vi "GetWorldPosition.vi"(8 "group":i32, 10 "Snpx":refnum<k24>, 11 "error in":errorcluster) -> (0 "UserTool":i16, 1 "Cartesian position":T1, 2 "JointsPosition":dbl[](array[numeric]), 3 "error out":errorcluster)   [LabVIEW 2015, in "UnderAutomation.Fanuc.lvlib"]
uses:
  UnderAutomation.Fanuc.lvlib
  C:/Users/fg/Documents/Fanuc.vi/LabVIEW_2024/UnderAutomation.Fanuc/lib/UnderAutomation.Fanuc.dll
  LabVIEW_2024/UnderAutomation.Fanuc/lib/UnderAutomation.Fanuc.dll
panel:
  out "UserFrame":i16
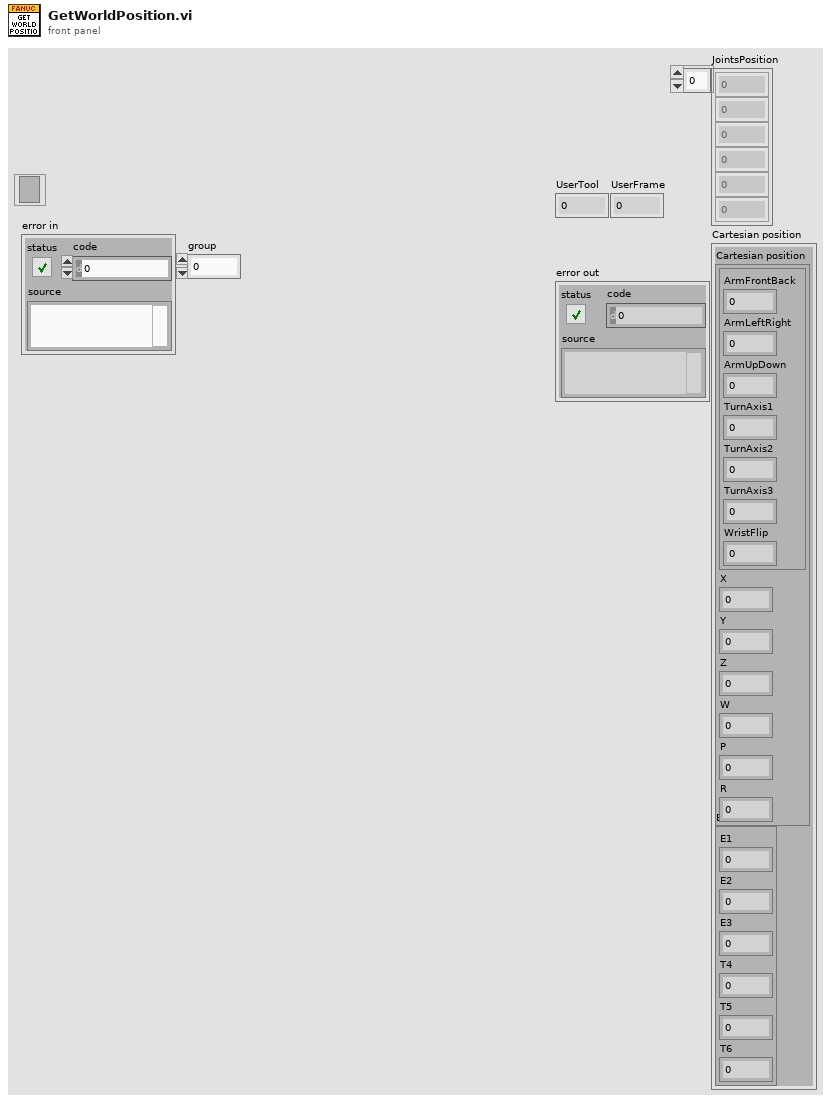
[diagram p1: front panel]
types:
  T1 = cluster{"Cartesian position":cluster{cluster{"ArmFrontBack":i32, "ArmLeftRight":i32, "ArmUpDown":i32, "TurnAxis1":i32, "TurnAxis2":i32, "TurnAxis3":i32, "WristFlip":i32}, "X":dbl, "Y":dbl, "Z":dbl, "W":dbl, "P":dbl, "R":dbl}, "Extension":cluster{"E1":dbl, "E2":dbl, "E3":dbl, "T4":i16, "T5":i16, "T6":i16}}
  T2 = cluster{"Configuration":cluster{"ArmFrontBack":i32, "ArmLeftRight":i32, "ArmUpDown":i32, "TurnAxis1":i32, "TurnAxis2":i32, "TurnAxis3":i32, "WristFlip":i32}, "X":dbl, "Y":dbl, "Z":dbl, "W":dbl, "P":dbl, "R":dbl}
  T3 = cluster{"E1":dbl, "E2":dbl, "E3":dbl, "E3":dbl, "E3":dbl, "E3":dbl}
  T4 = cluster{"Cartesian position":cluster{"Configuration":cluster{"ArmFrontBack":i32, "ArmLeftRight":i32, "ArmUpDown":i32, "TurnAxis1":i32, "TurnAxis2":i32, "TurnAxis3":i32, "WristFlip":i32}, "X":dbl, "Y":dbl, "Z":dbl, "W":dbl, "P":dbl, "R":dbl}, cluster{"E1":dbl, "E2":dbl, "E3":dbl, "E3":dbl, "E3":dbl, "E3":dbl}}
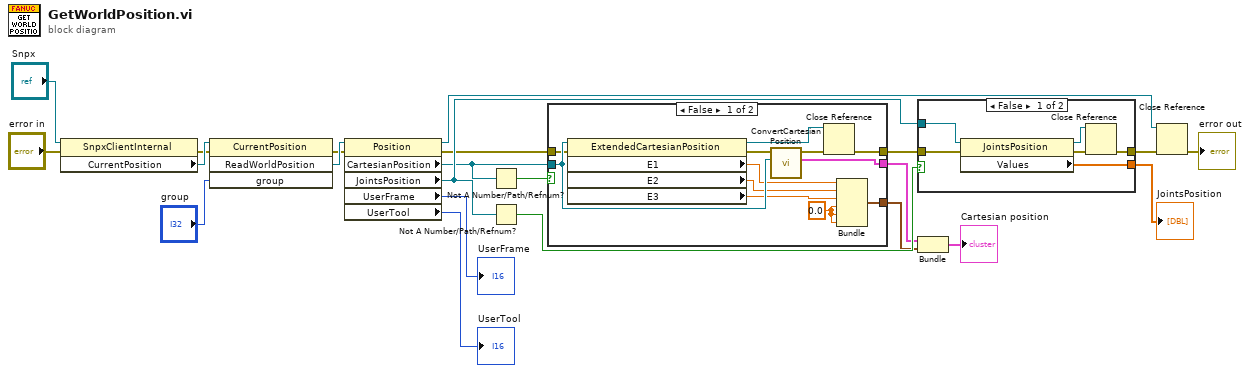
[diagram p0: block diagram]
diagram:
  n1 = property class="SnpxClientInternal"(reference="Snpx", error in="error in") -> (error out=w19:errorcluster, "CurrentPosition"=w20:refnum<k24>)  [unwired: 1 out]
  n2 = invoke class="CurrentPosition" method="ReadWorldPosition"(reference=w20, error in=w19, "group"="group") -> (error out=w3:errorcluster, "ReadWorldPosition"=w18:refnum<k24>)  [unwired: 1 in, 2 out]
  n3 = property class="Position"(reference=w18, error in=w3) -> (reference out=w17:refnum<k24>, error out=w6:errorcluster, "CartesianPosition"=w11:refnum<k24>, "JointsPosition"=w13:refnum<k24>, "UserFrame"=→"UserFrame":i16, "UserTool"=→"UserTool":i16)
  n4 = Not A Number/Path/Refnum?(number/path/refnum=w11) -> (NaN/Path/Refnum?=w10:bool)
  n5 = Not A Number/Path/Refnum?(number/path/refnum=w13) -> (NaN/Path/Refnum?=w14:bool)
  n6 = case shown="False" w10 {
    tunnel: w11 -> [w33 _]
    tunnel: [w34 _] -> w9
    tunnel: [w29 _] -> w8
    tunnel: w6 -> [w28 w35]
    tunnel: [w26 w35] -> w5
    frame False {
      w23 = 0.0 ("E3")
      n7 = property class="ExtendedCartesianPosition"(reference=w33, error in=w28) -> (reference out=w27:refnum<k24>, error out=w25:errorcluster, "E1"=w32:dbl, "E2"=w31:dbl, "E3"=w30:dbl)
      n8 = call "ConvertCartesianPosition.vi"("Cartesian position"=w33, "error in (no error)"=w25) -> ("Cartesian position"=w34:T2, "error out"=w24:errorcluster)  [unwired: 8 in]
      n9 = Close Reference(reference=w27, error in (no error)=w24) -> (error out=w26:errorcluster)
      n10 = Bundle("E1"=w32, "E2"=w31, "E3"=w30, "E3"=w23, "E3"=w23, "E3"=w23) -> (w29:T3)  [unwired: 1 in]
    }
    frame True {
    }
  }
  n11 = case shown="False" w14 {
    tunnel: w13 -> [w41 _]
    tunnel: [w40 _] -> w12
    tunnel: w5 -> [w37 w42]
    tunnel: [w36 w42] -> w4
    frame False {
      n12 = property class="JointsPosition"(reference=w41, error in=w37) -> (reference out=w38:refnum<k24>, error out=w39:errorcluster, "Values"=w40:dbl[])
      n13 = Close Reference(reference=w38, error in (no error)=w39) -> (error out=w36:errorcluster)
    }
    frame True {
    }
  }
  "JointsPosition" <- w12
  n14 = Bundle("Cartesian position"=w9, w8) -> (→"Cartesian position":T4)  [unwired: 1 in]
  n15 = Close Reference(reference=w17, error in (no error)=w4) -> (error out=→"error out":errorcluster)
